vi "Load Configuration.vi"(0 "INI Station Configuration in":refnum<class "Springboard Station Configuration.lvclass">, 5 "INI file path in":path, 11 "error in":errorcluster) -> (4 "INI Station Configuration out":refnum<class "Springboard Station Configuration.lvclass">, 15 "error out":errorcluster)   [LabVIEW 2018, in "Springboard TLB`.lvlib" / "Springboard Station Configuration.lvclass"]
uses:
  Springboard Station Configuration.lvclass
  Springboard Station Configuration.lvclass/Springboard Station Configuration.ctl
  <vilib>/Utility/config.llb/Read Key (String).vi
  <vilib>/Utility/config.llb/NI_LVConfig.lvlib
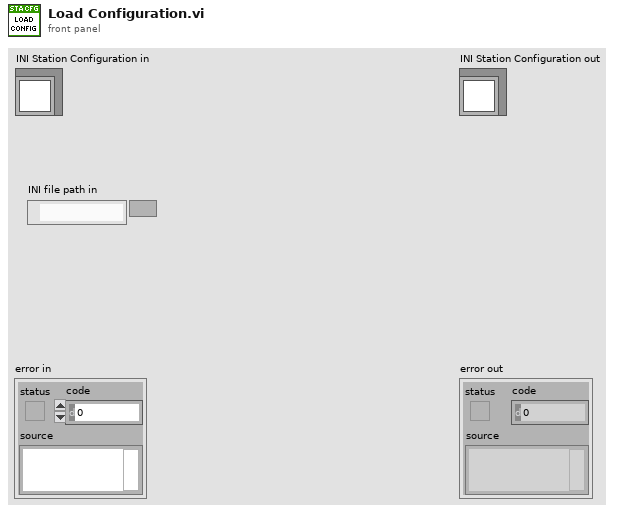
[diagram p1: front panel]
types:
  T1 = typedef "NI_LVConfig.lvlib/Config Data RefNum.ctl" = refnum<k1>
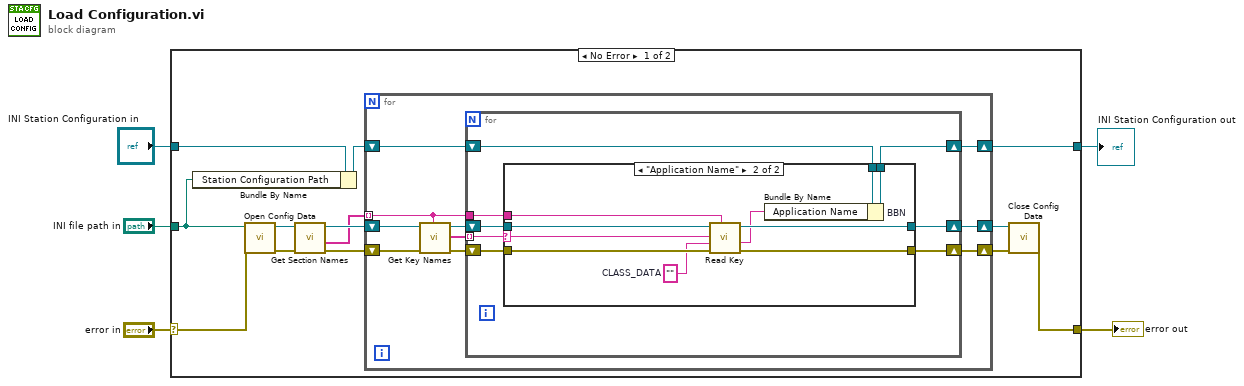
[diagram p0: block diagram]
diagram:
  n1 = case shown="No Error" "error in" {
    selector: "error in" -> [w17 w51]
    tunnel: [w18 w50] -> w2
    tunnel: [w14 w51] -> w1
    tunnel: "INI Station Configuration in" -> [w8 w50]
    tunnel: "INI file path in" -> [w6 _]
    frame No Error {
      n2 = Bundle By Name(cluster=w8, "Station Configuration Path"=w6) -> (w7:refnum<class "Springboard Station Configuration.lvclass">)
      n3 = call <vilib>:"Open Config Data.vi"("error in (no error)"=w17, "configuration file path"=w6) -> ("error out"=w11:errorcluster, "refnum"=w13:T1)  [unwired: 7 in, 1 out]
      n4 = call <vilib>:"Get Section Names.vi"("error in (no error)"=w11, "refnum"=w13) -> ("error out"=w9:errorcluster, "section names"=w10:string[], "refnum out"=w12:T1)  [unwired: 7 in]
      n5 = for {
        shift-right: [w28] -> w18
        shift-left: w7 -> [w27]
        shift-right: [w24] -> w15
        shift-left: w9 -> [w20]
        shift-right: [w25] -> w16
        shift-left: w12 -> [w26]
        tunnel: w10 -> [w22] mode=indexing
        n6 = call <vilib>:"Get Key Names.vi"("section"=w22, "error in (no error)"=w20, "refnum"=w26) -> ("error out"=w19:errorcluster, "key names"=w21:string[], "refnum out"=w23:T1)  [unwired: 5 in, 1 out]
        n7 = for {
          shift-right: [w36] -> w28
          shift-left: w27 -> [w31]
          shift-right: [w33] -> w24
          shift-left: w19 -> [w35]
          shift-right: [w32] -> w25
          shift-left: w23 -> [w34]
          tunnel: w22 -> [w30]
          tunnel: w21 -> [w29] mode=indexing
          n8 = case shown="\"Application Name\"" w29 {
            selector: w29 -> [_ w40]
            tunnel: [w37 w43] -> w36
            tunnel: w35 -> [w38 w48]
            tunnel: w34 -> [w39 w49]
            tunnel: [w38 w46] -> w33
            tunnel: [w39 w45] -> w32
            tunnel: w31 -> [w37 w41]
            tunnel: w30 -> [_ w42]
            frame Default {
            }
            frame "Application Name" {
              w47 = ""  # CLASS_DATA
              n9 = call-poly <vilib>:"Read Key.vi"("section"=w42, "error in (no error)"=w48, "default value"=w47, "key"=w40, "refnum"=w49) -> ("error out"=w46:errorcluster, "value"=w44:string, "refnum out"=w45:T1)  [unwired: 3 in, 1 out]
              n10 = Bundle By Name "BBN"(cluster=w41, "Application Name"=w44) -> (w43:refnum<class "Springboard Station Configuration.lvclass">)
            }
          }
        }
      }
      n11 = call <vilib>:"Close Config Data.vi"("error in (no error)"=w15, "refnum"=w16) -> ("error out"=w14:errorcluster)  [unwired: 8 in, 1 out]
    }
    frame Error {
    }
  }
  "error out" <- w1
  "INI Station Configuration out" <- w2
